vi "Write Build Directory.vi"(5 "Build Directory":path, 9 "PythonConverter_BD in":refnum<class "PythonBDConverter.lvclass">) -> (3 "PythonConverter_BD out":refnum<class "PythonBDConverter.lvclass">)   [LabVIEW 2014, in "PythonBDConverter.lvclass"]
uses:
  PythonBDConverter.lvclass
  PythonBDConverter.lvclass/PythonBDConverter.ctl
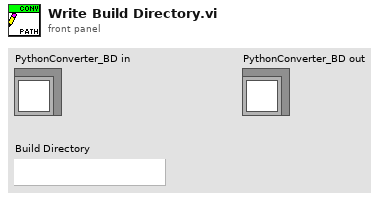
[diagram p1: front panel]
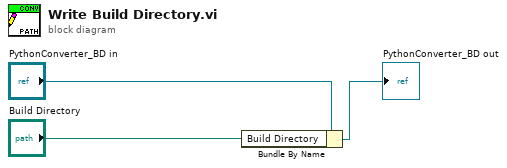
[diagram p0: block diagram]
diagram:
  n1 = Bundle By Name(cluster="PythonConverter_BD in", "Build Directory"="Build Directory") -> (→"PythonConverter_BD out":refnum<class "PythonBDConverter.lvclass">)
